vi "crd_Acquire.vi"() -> ()   [LabVIEW 2011]
panel:
  in  "No Avg.":i32=1 min=1
  out "Decay":cluster{sgl[], "Best Exponential Fit":dbl[]}[](graph)
  out "error out":errorcluster
  out "Tau vs. T":dbl(graph)
  in  "stop":bool
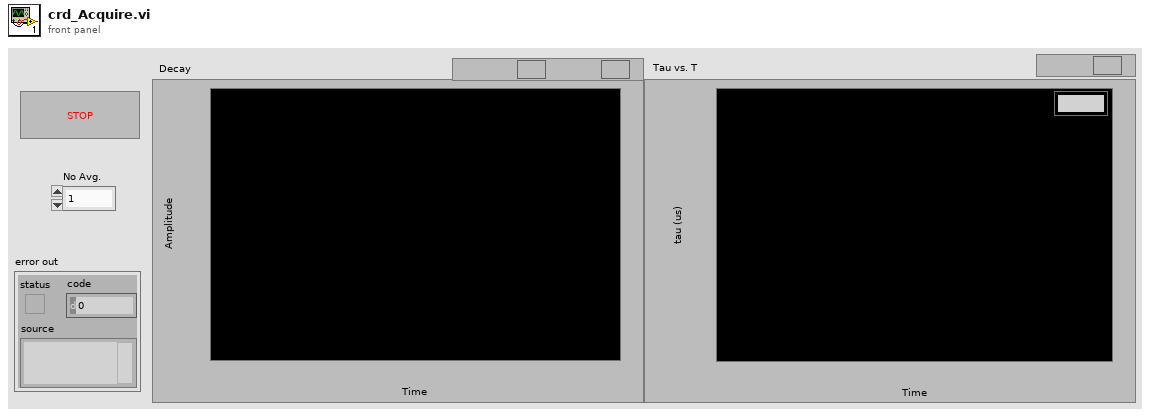
[diagram p1: front panel]
types:
  T1 = cluster{i32, "Sample Internal":sgl, "Data (Volts)":dbl[]}
  T2 = cluster{"Driver Version":string, "USB Version":string, "Hardware":string, "Variant":string, "Batch and Serial":string, "Cal Date":string, "Kernel Version":string, "Digital HW Version":string, "Analogue HW Version":string, "Firmware 1":string, "Firmware 2":string, "MSO":bool, "Number of Channels":i16}
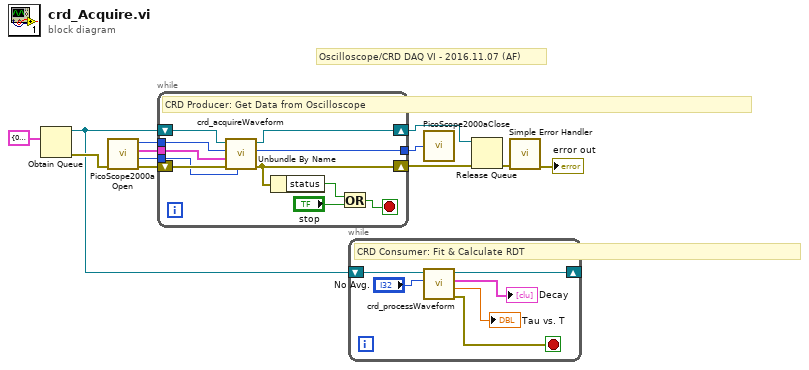
[diagram p0: block diagram]
diagram:
  # "Oscilloscope/CRD DAQ VI - 2016.11.07 (AF)"
  n1 = Obtain Queue(element data type=T1 {0, "Sample Internal"=8e-09, "Data (Volts)"=array[20000 elements]} ("Channel A 2")) -> (queue out=w4:refnum<queue>, error out=w7:errorcluster)  [unwired: 4 in, 1 out]
  n2 = call "PicoScope2000aOpen.vi"("error in (no error)"=w7) -> ("error out"=w11:errorcluster, "Max Adc value"=w12:i16, "Device Info"=w10:T2, "handle"=w9:i16)  [unwired: 7 in]
  n3 = while {
    tunnel: w10 -> [w19]
    tunnel: w9 -> [w20]
    tunnel: w12 -> [w14]
    tunnel: [w17] -> w3
    shift-right: [w16] -> w6
    shift-left: w4 -> [w15]
    shift-right: [w13] -> w5
    shift-left: w11 -> [w21]
    stop <- w22 stop-if-true
    # "CRD Producer: Get Data from Oscilloscope"
    n4 = call "crd_acquireWaveform.vi"("Max Adc value"=w14, "error in (no error)"=w21, "Device Info"=w19, "handle"=w20, "Queue in"=w15) -> ("error out"=w13:errorcluster, "handle out"=w17:i16, "Queue out"=w16:refnum<queue>)  [unwired: 4 in]
    n5 = Unbundle By Name(w13) -> ("status"=w18:bool)
    n6 = Or(x=w18, y="stop") -> (x .or. y?=w22:bool)
  }
  n7 = while {
    shift-right: [w25] -> _
    shift-left: w4 -> [w26]
    stop <- w24 stop-if-true
    # "CRD Consumer: Fit & Calculate RDT"
    n8 = call "crd_processWaveform.vi"("No Avg."="No Avg.", "Queue in"=w26) -> ("error out"=w24:errorcluster, "tau (us)"=→"Tau vs. T":dbl, "Decay"=→"Decay":cluster{sgl[], "Best Exponential Fit":dbl[]}[], "Queue out"=w25:refnum<queue>)  [unwired: 6 in]
  }
  n9 = call "PicoScope2000aClose.vi"("handle"=w3) -> ()
  n10 = Release Queue(queue=w6, error in (no error)=w5) -> (error out=w1:errorcluster)  [unwired: 1 in, 2 out]
  n11 = call <vilib>:"Simple Error Handler.vi"("error in (no error)"=w1) -> ("error out"=→"error out":errorcluster)  [unwired: 4 in, 4 out]
